vi "UDP_receiveAndSendBack.vi"() -> ()   [LabVIEW 2021]
panel:
  out "error out":errorcluster
  in  "stop":bool
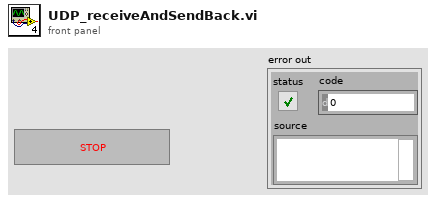
[diagram p1: front panel]
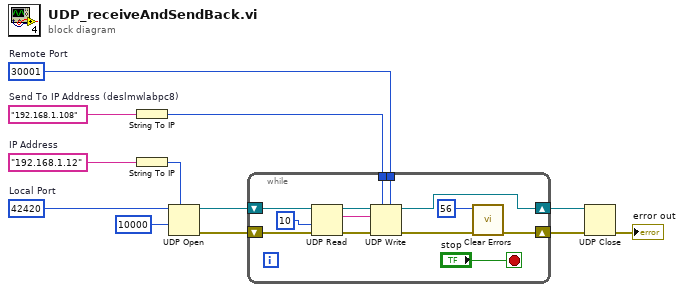
[diagram p0: block diagram]
diagram:
  w1 = u16 42420  # Local Port
  w2 = "192.168.1.12"  # IP Address
  w3 = u16 30001  # Remote Port
  w4 = "192.168.1.108"  # Send To IP Address (deslmwlabpc8)
  n1 = String To IP(1:w4) -> (0:w8:u32)
  n2 = String To IP(1:w2) -> (0:w9:u32)
  n3 = UDP Open(7:w9, 9:10000 ("timeout ms (25000)"), 11:w1) -> (port=w11:refnum<k16>, 0:w10:errorcluster)  [unwired: 2 in, 1 out]
  n4 = while {
    tunnel: w8 -> [w19]
    shift-right: [w17] -> w6
    shift-left: w10 -> [w23]
    shift-right: [w15] -> w7
    shift-left: w11 -> [w25]
    tunnel: w3 -> [w13]
    stop <- "stop" stop-if-true
    n5 = UDP Read(connection ID=w25, timeout ms (25000)=10, 8:w23) -> (data out=w21:string, error out=w20:errorcluster, 3:w22:refnum<k16>)  [unwired: 1 in, 2 out]
    n6 = UDP Write(address=w19, port or service name=w13, connection ID=w22, data in=w21, 8:w20) -> (error out=w16:errorcluster, 3:w15:refnum<k16>)  [unwired: 1 in]
    n7 = call <vilib>:"Clear Errors.vi"("error in (no error)"=w16, "specific error code to clear (0: all)"=56) -> ("error out"=w17:errorcluster)  [unwired: 4 in, 1 out]
  }
  n8 = UDP Close(connection ID=w7, 8:w6) -> (error out=→"error out":errorcluster)  [unwired: 1 out]
